vi "Configure Acquisition Type.vi"(8 "error in (no error)":errorcluster, 10 "acquisition type (Normal)":i32(ring) items=["Normal", "Peak Detect", "High Resolution", "Envelope", "Average"], 11 "CS++Scope":refnum<class "CS++Scope.lvclass">) -> (0 "error out":errorcluster, 3 "CS++Scope out":refnum<class "CS++Scope.lvclass">)   [LabVIEW 2014, in "CS++Scope.lvlib" / "CS++Scope.lvclass"]
doc: "This VI configures how the oscilloscope acquires data and how it fills the waveform record."
uses:
  CS++Scope.lvclass
  CSPP_Core/Classes/CS++ProcessVariables/ProcessVariable/PV.lvclass
  PV-Enum.ctl
  CSPP_Core/Classes/CS++ProcessVariables/ProcessVariable/PV.lvclass/PV.ctl
  CS++Scope.lvclass/CS++Scope.ctl
  CSPP_Core/Classes/CS++ProcessVariables/ProcessVariable/Write Data.vi
  CSPP_Core/Classes/CS++ProcessVariables/ProcessVariable/Write Timestamp.vi
  CSPP_Core/Classes/CS++ProcessVariables/ProcessVariable/Write Quality.vi
  CSPP_Core/Classes/CS++ProcessVariables/ProcessVariable/Write status.vi
  CSPP_Core/Classes/CS++ProcessVariables/PVConnection/PVConnection.lvclass
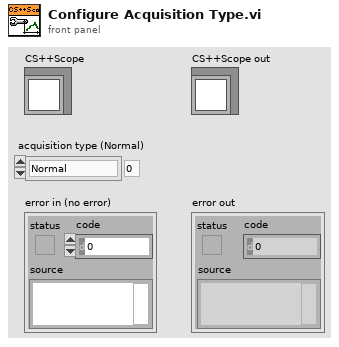
[diagram p1: front panel]
types:
  T1 = typedef "CS++Scope.lvlib/CS++Scope.lvclass/PV-Enum.ctl" = enum16{"ActualSampleRate", "TimePerRecord", "AcquisitionStartTime", "TriggerLevel", "GlitchWidth", "LowReference", "MidReference", "HighReference", "RuntLowThreshold", "RuntHighThreshold", "TriggerHoldoff", "WidthLowThreshold", "WidthHighThreshold", "AcquisitionStatus", "ActualRecordLength", "ActualSampleMode", "ACLineTriggerSlope", "MinRecordLength", "AcquisitionType", "TriggerSlope", "GlitchCondition", "GlitchPolarity", "InterpolationMethod", "NumberOfAverages", "NumberOfEnvelopes", "TriggerType", "TriggerCoupling", "TriggerModifier", "TVLineNumber", "TVEvent", "TVTriggerPolarity", "TVSignalFormat", "WidthCondition", "WidthPolarity", "MeasurementDone", "ContinousAcquisition", "TriggerSource", "Waveform", "ActualTimeIncrement"}
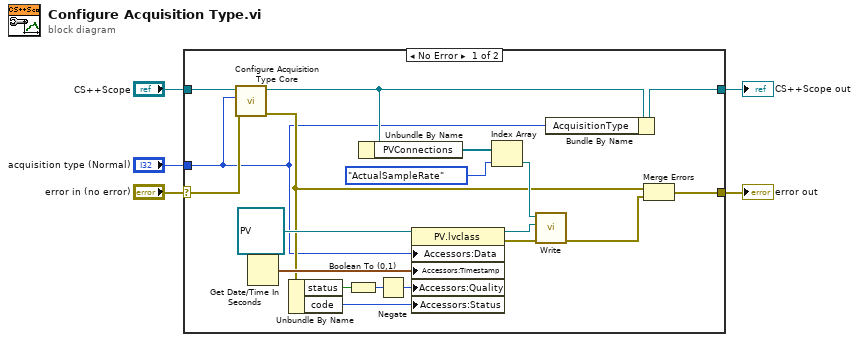
[diagram p0: block diagram]
diagram:
  n1 = case shown="No Error" "error in (no error)" {
    selector: "error in (no error)" -> [w23 w26]
    tunnel: [w7 w26] -> w4
    tunnel: [w21 w25] -> w2
    tunnel: "CS++Scope" -> [w24 w25]
    tunnel: "acquisition type (Normal)" -> [w6 _]
    frame No Error {
      n2 = call-dynamic "Configure Acquisition Type Core.vi"("error in (no error)"=w23, "acquisition type (Normal)"=w6, "CS++Scope"=w24) -> ("error out"=w9:errorcluster, "CS++Scope out"=w22:refnum<class "CS++Scope.lvclass">)  [unwired: 7 in]
      n3 = Get Date/Time In Seconds() -> (seconds since 1Jan1904=w15:timestamp)
      n4 = Unbundle By Name(w9) -> ("status"=w18:bool, "code"=w19:i32)
      n5 = Boolean To (0,1)(Boolean=w18) -> (0, 1=w17:i16)
      n6 = Unbundle By Name(w22) -> ("PVConnections"=w12:refnum<class "PVConnection.lvclass">[])
      n7 = Negate(x=w17) -> (-x=w16:i16)
      n8 = property class="PV.lvclass"(reference=refnum<class "PV.lvclass"> refnum ("CS++ProcessVariables.lvlib:PV.lvclass"), "Accessors:Data"=w6, "Accessors:Timestamp"=w15, "Accessors:Quality"=w16, "Accessors:Status"=w19) -> (reference out=w14:refnum<class "PV.lvclass">, error out=w13:errorcluster)  [unwired: 1 in]
      n9 = Index Array(array=w12, index=PV-Enum."ActualSampleRate" ("PV-Enum")) -> (element=w10:refnum<class "PVConnection.lvclass">)
      n10 = call "Write.vi"("error in (no error)"=w13, "PV"=w14, "PVConnection in"=w10) -> ("error out"=w8:errorcluster)  [unwired: 7 in, 1 out]
      n11 = Bundle By Name(cluster=w22, "AcquisitionType"=w6) -> (w21:refnum<class "CS++Scope.lvclass">)
      n12 = Merge Errors(w9, w8) -> (w7:errorcluster)
    }
    frame Error {
    }
  }
  "error out" <- w4
  "CS++Scope out" <- w2
